vi "Execute.vi"(8 "error in":errorcluster, 10 "Stop CMD in":refnum<class "Stop CMD.lvclass">, 11 "Instrument In":refnum<class>) -> (0 "error out":errorcluster, 3 "Instrument Out":refnum<class>)   [LabVIEW 2014, in "Instrument.lvlib" / "Stop CMD.lvclass"]
doc: "Set the new Instrument object state to Quit."
uses:
  Stop CMD.lvclass
  Instrument.lvclass
  state.ctl
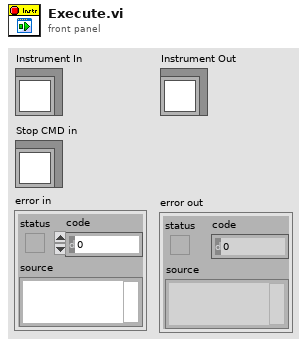
[diagram p1: front panel]
types:
  T1 = typedef "Instrument.lvclass/state.ctl" = enum8{"Configure", "Acquire", "Wait", "Quit", "Handle Error", "NOOP"}
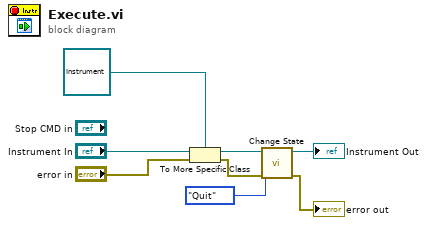
[diagram p0: block diagram]
diagram:
  n1 = To More Specific Class(target class=refnum<class "Instrument.lvclass"> refnum ("Instrument.lvclass"), reference="Instrument In", error in="error in") -> (specific class reference=w6:refnum<class "Instrument.lvclass">, error out=w2:errorcluster)
  n2 = call "Change State.vi"("error in"=w2, "instr state"=state."Quit", "Instrument in"=w6) -> ("error out"=→"error out":errorcluster, "Instrument out"=→"Instrument Out":refnum<class "Instrument.lvclass">)  [unwired: 7 in]
